vi "uActor_HandlErr.vi"(8 "error in (no error)":errorcluster, 11 "uActor in":refnum<class "uActor.lvclass">) -> (0 "error out":errorcluster, 3 "uActor out":refnum<class "uActor.lvclass">)   [LabVIEW 2023, in "uLib.lvlib" / "uActor.lvclass"]
doc: "Protected method that wraps the uErr.Handle method.\nThe actor will stop if the error is not cleared by the runtime's uErr object.\n\nThis protected method is made available for the use in helper loops if required; to give them the same error handling behavior as the actor core loop."
uses:
  uActor.lvclass
  uActor.lvclass/uActor.ctl
  uErr/uErr/uErr.lvclass
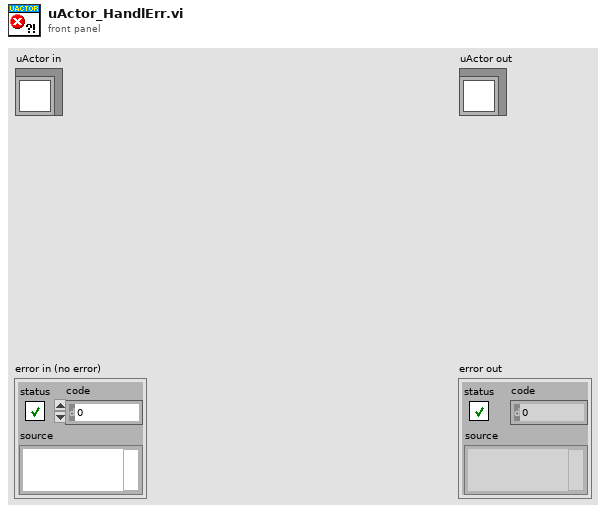
[diagram p1: front panel]
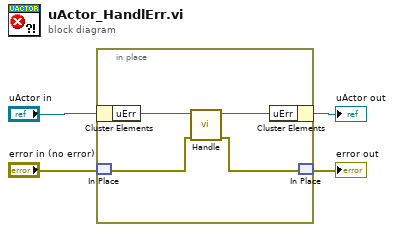
[diagram p0: block diagram]
diagram:
  n1 = in-place {
    n2 = in-place-cluster #1("uActor in") -> ("uErr"=w8:refnum<class "uErr.lvclass">)
    n3 = in-place-match #2("error in (no error)") -> (w6:errorcluster)
    n4 = call-dynamic "Handle.vi"("error in (no error)"=w6, "uErr in"=w8) -> ("error out"=w5:errorcluster, "uErr out"=w7:refnum<class "uErr.lvclass">)  [unwired: 8 in]
    n5 = in-place-cluster #1("uErr"=w7) -> (→"uActor out":refnum<class "uActor.lvclass">)
    n6 = in-place-match #2(w5) -> (→"error out":errorcluster)
  }
